vi "spill_param_tcp_query.vi"(0 "n_try":i32=2, 3 "time_out":i32=100) -> (7 "spill_id":i32=-1, 10 "status":bool=TRUE)   [LabVIEW 2019]
panel:
  out "client_step":i32
  out "error out":errorcluster
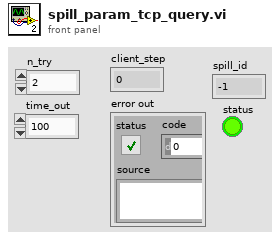
[diagram p1: front panel]
types:
  T1 = enum16{"Standard", "Buffered", "CRLF", "Immediate"}
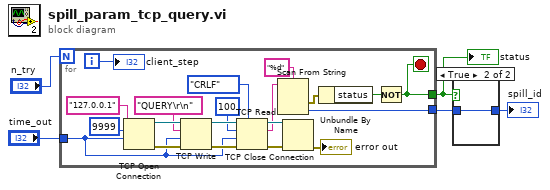
[diagram p0: block diagram]
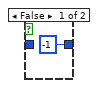
[diagram p2: hidden frame]
diagram:
  n1 = for {
    N: "n_try" -> [_]
    tunnel: "time_out" -> [w6]
    tunnel: [w7] -> w1
    tunnel: [w9] -> w2
    i -> [w10]
    stop <- w7 stop-if-true
    n2 = TCP Open Connection(address="127.0.0.1", remote port or service name=u16 9999, timeout ms (60000)=w6) -> (connection ID=w23:refnum<k5>, error out=w22:errorcluster)  [unwired: 2 in]
    n3 = TCP Write(connection ID=w23, data in="QUERY\r\n", error in (no error)=w22, 9:w6) -> (connection ID out=w19:refnum<k5>, error out=w20:errorcluster)  [unwired: 1 out]
    n4 = TCP Read(connection ID=w19, bytes to read=100, error in (no error)=w20, 7:T1."CRLF" ("mode (standard)"), 9:w6) -> (connection ID out=w17:refnum<k5>, data out=w15:string, error out=w18:errorcluster)
    n5 = Scan From String(format string="%d", input string=w15) -> (error out=w13:errorcluster, output 1=w9:i32)  [unwired: 3 in, 2 out]
    n6 = TCP Close Connection(connection ID=w17, error in (no error)=w18) -> (error out=→"error out":errorcluster)  [unwired: 1 in, 1 out]
    n7 = Unbundle By Name(w13) -> ("status"=w8:bool)
    n8 = Not(x=w8) -> (.not. x?=w7:bool)
    "client_step" <- w10
  }
  "status" <- w1
  n9 = case shown="True" w1 {
    tunnel: [-1 w27] -> w3
    tunnel: w2 -> [_ w27]
    frame False {
    }
    frame True {
    }
  }
  "spill_id" <- w3
